vi "AutoFocus.vi"(7 "Start Z":dbl, 8 "error in":errorcluster, 9 "Range(mm)":dbl=0.2, 10 "Steps":i32=10, 11 "CameraTool Class In":refnum<class "CameraTool Class.lvclass">) -> (0 "error out":errorcluster, 2 "focus height":dbl, 3 "CameraTool Class Out":refnum<class "CameraTool Class.lvclass">)   [LabVIEW 2011, in "CameraTool Class.lvclass"]
doc: "This VI returns the \"variance of laplacians\" measure of image focus."
uses:
  CameraTool Class.lvclass
  Config Manager Class/Type Definitions/Camera Enum.ctl
  Vec3d Class/Vec3d Class.lvclass
  gVision API/gVision/gVision.lvlib
panel:
  out "XY Graph":cluster{"X":dbl, "Y":dbl}[](graph)
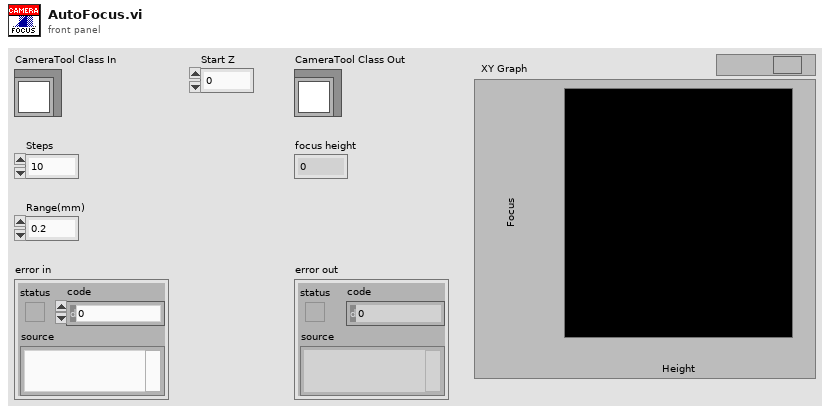
[diagram p1: front panel]
types:
  T1 = typedef "Camera Enum.ctl" = enum16{"GANTRY HEAD", "NEEDLE CALIBRATION X", "NEEDLE CALIBRATION Y"}
  T2 = typedef "IMAQ Image.ctl" = refnum<image>
  T3 = typedef "Physical Image.ctl" = cluster{"Image Position":refnum<class "Vec3d Class.lvclass">, "Image Reference":T2, "Field of View":cluster{"x(mm)":dbl, "y(mm)":dbl}}
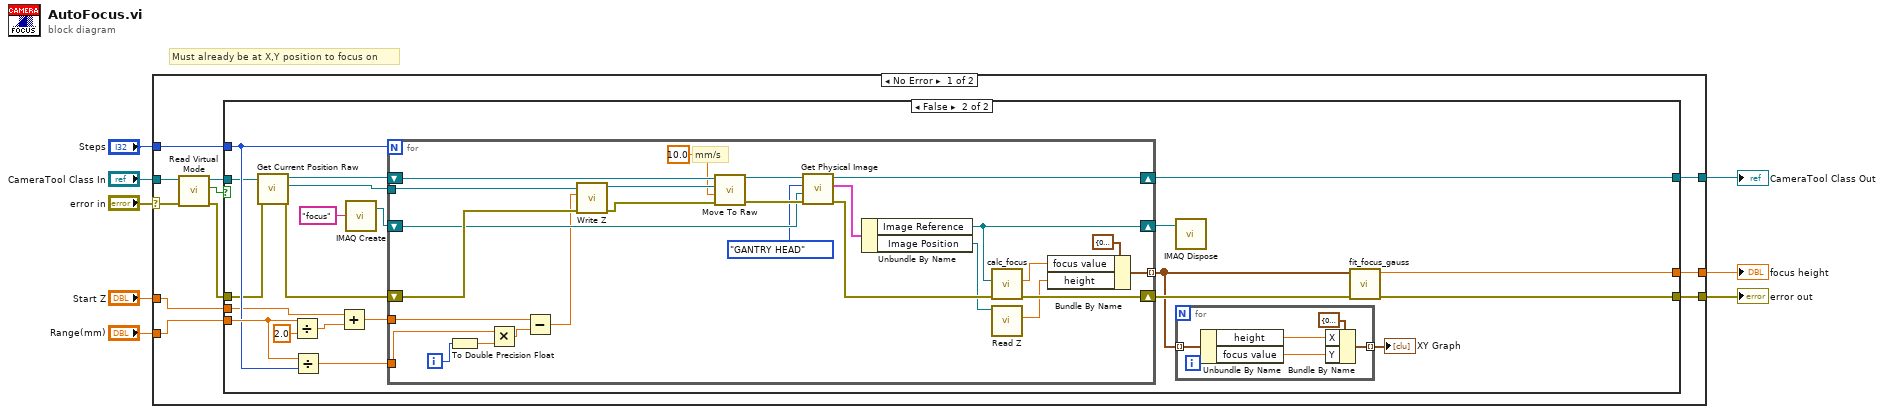
[diagram p0: block diagram]
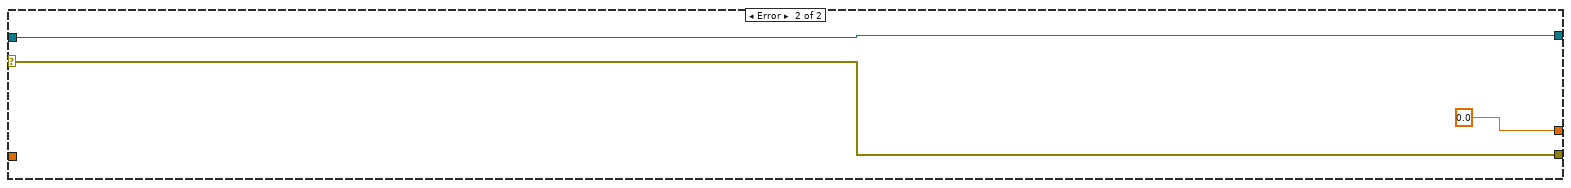
[diagram p3: hidden frame]
diagram:
  # "Must already be at X,Y position to focus on"
  n1 = case shown="No Error" "error in" {
    selector: "error in" -> [w11 w75]
    tunnel: "Start Z" -> [w14 _]
    tunnel: "CameraTool Class In" -> [w13 w77]
    tunnel: [w17 sgl 0.0 ("return type")] -> w5
    tunnel: [w18 w75] -> w4
    tunnel: [w19 w77] -> w3
    tunnel: "Steps" -> [w15 _]
    tunnel: "Range(mm)" -> [w16 _]
    frame No Error {
      n2 = call-dynamic "Read Virtual Mode.vi"("error in (no error)"=w11, "Gantry Class in"=w13) -> ("error out"=w9:errorcluster, "Virtual Mode"=w10:bool, "Gantry Class out"=w12:refnum<class "CameraTool Class.lvclass">)  [unwired: 7 in]
      n3 = case shown="False" w10 {
        tunnel: [w22 w42] -> w19
        tunnel: [w21 w25] -> w18
        tunnel: [w20 w27] -> w17
        tunnel: w16 -> [_ w38]
        tunnel: w15 -> [_ w37]
        tunnel: w14 -> [w20 w34]
        tunnel: w12 -> [w22 w29]
        tunnel: w9 -> [w21 w28]
        frame True {
        }
        frame False {
          n4 = call-dynamic "Get Current Position Raw.vi"("error in"=w28, "Gantry in"=w29) -> ("error out"=w40:errorcluster, "Vec3d Class out"=w43:refnum<class "Vec3d Class.lvclass">, "Gantry out"=w41:refnum<class "CameraTool Class.lvclass">)  [unwired: 7 in]
          n5 = Divide(x=w38, y=2.0) -> (x/y=w35:dbl)
          n6 = Divide(x=w38, y=w37) -> (x/y=w36:dbl)
          n7 = Add(x=w34, y=w35) -> (x+y=w33:dbl)
          n8 = call "IMAQ Create"("Image Name"="focus") -> ("New Image"=w31:T2)  [unwired: 4 in, 1 out]
          n9 = for {
            N: w37 -> [_]
            tunnel: w43 -> [w72]
            shift-right: [w66] -> w42
            shift-left: w41 -> [w73]
            shift-right: [w65] -> w26
            shift-left: w40 -> [w70]
            tunnel: w36 -> [w64]
            tunnel: w33 -> [w63]
            shift-right: [w51] -> w30
            shift-left: w31 -> [w60]
            tunnel: [w55] -> w24 mode=indexing
            i -> [w62]
            # "mm/s"
            n10 = To Double Precision Float(number=w62) -> (double precision float=w61:dbl)
            n11 = Multiply(x=w64, y=w61) -> (x*y=w74:dbl)
            n12 = Subtract(x=w63, y=w74) -> (x-y=w56:dbl)
            n13 = call-dynamic "Write Z.vi"("error in (no error)"=w70, "Z"=w56, "Vec3d Class in"=w72) -> ("error out"=w69:errorcluster, "Vec3d Class out"=w71:refnum<class "Vec3d Class.lvclass">)  [unwired: 7 in]
            n14 = call-dynamic "Move To Raw.vi"("error in"=w69, "Speed"=10.0, "Destination"=w71, "Gantry in"=w73) -> ("error out"=w67:errorcluster, "Gantry out"=w68:refnum<class "CameraTool Class.lvclass">)  [unwired: 6 in]
            n15 = call-dynamic "Get Physical Image.vi"("error in"=w67, "Image In"=w60, "Camera Name"=Camera_Enum."GANTRY HEAD", "Gantry in"=w68) -> ("error out"=w59:errorcluster, "Physical Image"=w52:T3, "Gantry out"=w66:refnum<class "CameraTool Class.lvclass">)  [unwired: 5 in]
            n16 = Unbundle By Name(w52) -> ("Image Reference"=w51:T2, "Image Position"=w50:refnum<class "Vec3d Class.lvclass">)
            n17 = call "calc_focus.vi"("error in"=w59, "Image"=w51) -> ("error out"=w65:errorcluster, "focus"=w57:sgl)  [unwired: 7 in, 1 out]
            n18 = call-dynamic "Read Z.vi"("Vec3d Class in"=w50) -> ("Z"=w49:dbl)  [unwired: 8 in, 2 out]
            n19 = Bundle By Name(cluster=cluster{"focus value":dbl, "height":dbl} {"focus value"=0.0, "height"=0.0} ("Focus Measurement"), "focus value"=w57, "height"=w49) -> (w55:cluster{"focus value":dbl, "height":dbl})
          }
          n20 = call "IMAQ Dispose"("Image"=w30) -> ()  [unwired: 5 in, 1 out]
          n21 = for {
            tunnel: w24 -> [w48] mode=indexing
            tunnel: [w44] -> w23 mode=indexing
            n22 = Unbundle By Name(w48) -> ("height"=w46:dbl, "focus value"=w45:dbl)
            n23 = Bundle By Name(cluster=cluster{"X":dbl, "Y":dbl} {"X"=0.0, "Y"=0.0}, "X"=w46, "Y"=w45) -> (w44:cluster{"X":dbl, "Y":dbl})
          }
          "XY Graph" <- w23
          n24 = call "fit_focus_gauss.vi"("error in"=w26, "Focus Measurements"=w24) -> ("error out"=w25:errorcluster, "focus height"=w27:dbl)  [unwired: 7 in, 1 out]
        }
      }
    }
    frame Error {
    }
  }
  "CameraTool Class Out" <- w3
  "error out" <- w4
  "focus height" <- w5
